vi "Delete Policy Version.vi"(8 "error in (no error)":errorcluster, 9 "Version":i32, 10 "Name":string, 11 "IoT Session in":refnum<class "IoT Session.lvclass">) -> (0 "error out":errorcluster, 3 "IoT Session out":refnum<class "IoT Session.lvclass">)   [LabVIEW 2015, in "NI_AWS_IoT.lvlib" / "IoT Session.lvclass"]
uses:
  IoT Session.lvclass
  Core/HTTP Request/Request Options.ctl
  Core/HTTP Request/Name Value Pair.ctl
  Core/HTTP Request/Region handling.ctl
  Core/HTTP Request/URL formatting.ctl
  Core/HTTP Request/HTTP Request.lvclass
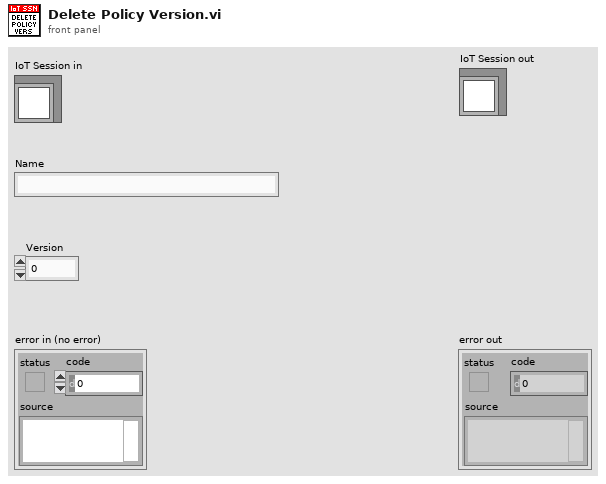
[diagram p1: front panel]
types:
  T1 = typedef "NI_AWS_Core.lvlib/HTTP Request.lvclass/Name Value Pair.ctl" = cluster{"name":string, "value":string}
  T2 = typedef "NI_AWS_Core.lvlib/HTTP Request.lvclass/Request Options.ctl" = cluster{"request headers":T1[], "request parameters":T1[], "request body":string, "region handling":T3, "URL formatting":T4}
  T3 = typedef "NI_AWS_Core.lvlib/HTTP Request.lvclass/Region handling.ctl" = enum16{"use region everywhere", "use region (authentication only)", "use region (URL only)", "ignore region everwhere"}
  T4 = typedef "NI_AWS_Core.lvlib/HTTP Request.lvclass/URL formatting.ctl" = enum16{"region-", "region."}
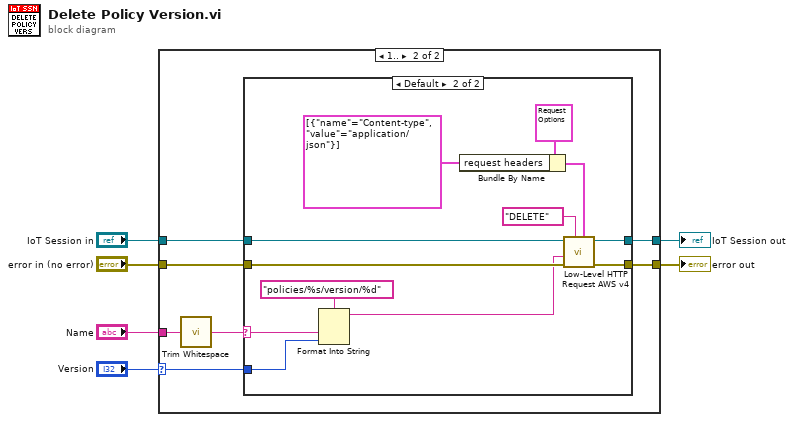
[diagram p0: block diagram]
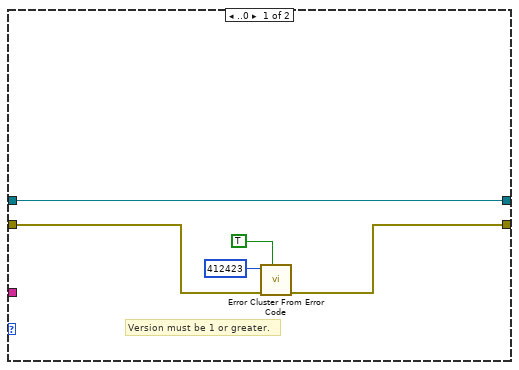
[diagram p2: hidden frame]
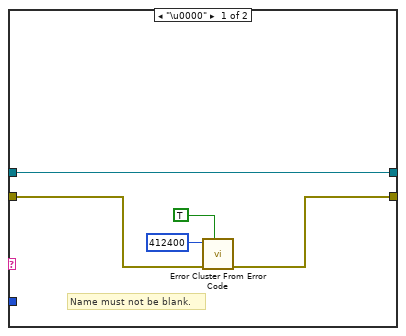
[diagram p3: hidden frame]
diagram:
  n1 = case shown="1.." "Version" {
    selector: "Version" -> [_ w12]
    tunnel: "error in (no error)" -> [w10 w18]
    tunnel: [w9 w17] -> w5
    tunnel: [w11 w16] -> w4
    tunnel: "Name" -> [_ w15]
    tunnel: "IoT Session in" -> [w11 w14]
    frame ..0 {
      # "Version must be 1 or greater."
      n2 = call <vilib>:"Error Cluster From Error Code.vi"("show call chain? (False)"=TRUE, "error in (no error)"=w10, "error code (0)"=412423) -> ("error out"=w9:errorcluster)  [unwired: 6 in]
    }
    frame 1.. {
      n3 = call <vilib>:"Trim Whitespace.vi"("string"=w15) -> ("trimmed string"=w13:string)  [unwired: 1 in]
      n4 = case shown="Default" w13 {
        selector: w13 -> [_ w31]
        tunnel: w18 -> [w20 w35]
        tunnel: [w19 w34] -> w17
        tunnel: [w23 w33] -> w16
        tunnel: w14 -> [w23 w32]
        tunnel: w12 -> [_ w24]
        frame "\u0000" {
          # "Name must not be blank."
          n5 = call <vilib>:"Error Cluster From Error Code.vi"("show call chain? (False)"=TRUE, "error in (no error)"=w20, "error code (0)"=412400) -> ("error out"=w19:errorcluster)  [unwired: 6 in]
        }
        frame Default {
          n6 = Format Into String(format string="policies/%s/version/%d", w31, w24) -> (resulting string=w28:string)  [unwired: 2 in, 1 out]
          n7 = Bundle By Name(cluster=T2 {"request headers"=[], "request parameters"=[], "request body"="", "region handling"=enum."use region everywhere", "URL formatting"=enum."region."} ("Request Options"), "request headers"=T1[] [{"name"="Content-type", "value"="application/json"}]) -> (w26:T2)
          n8 = call "Low-Level HTTP Request AWS v4.vi"("Request Options"=w26, "HTTP-Verb"="DELETE", "error in (no error)"=w35, "URL Suffix"=w28, "AWS Core in"=w32) -> ("error out"=w34:errorcluster, "AWS Core out"=w33:refnum<class "IoT Session.lvclass">)  [unwired: 3 in, 2 out]
        }
      }
    }
  }
  "error out" <- w5
  "IoT Session out" <- w4
